vi "Check Protection.vi"(8 "error in (no error)":errorcluster, 10 "String in":string, 11 "LRC - HRZ Series in":refnum<class "LRC - HRZ Series.lvclass">) -> (0 "error out":errorcluster, 1 "Protection Error":errorcluster, 2 "String out":string, 3 "LRC - HRZ Series out":refnum<class "LRC - HRZ Series.lvclass">)   [LabVIEW 2020, in "Protections.lvlib" / "LRC - HRZ Series.lvclass"]
uses:
  LRC - HRZ Series.lvclass
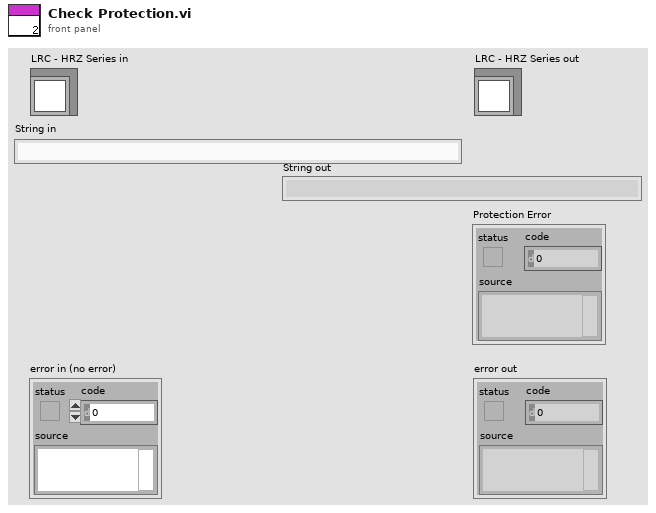
[diagram p1: front panel]
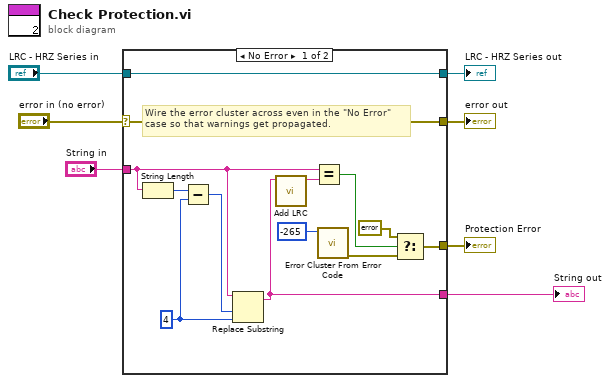
[diagram p0: block diagram]
diagram:
  n1 = case shown="No Error" "error in (no error)" {
    selector: "error in (no error)" -> [w19 w23]
    tunnel: [w19 w23] -> w6
    tunnel: [w20 w22] -> w4
    tunnel: "LRC - HRZ Series in" -> [w20 w22]
    tunnel: "String in" -> [w14 w21]
    tunnel: [w9 _] -> w2
    tunnel: [w8 w21] -> w1
    frame No Error {
      w16 = 4
      # "Wire the error cluster across even in the \"No Error\"\ncase so that warnings get propagated."
      n2 = String Length(string=w14) -> (length=w18:i32)
      n3 = Subtract(x=w18, y=w16) -> (x-y=w17:i32)
      n4 = Replace Substring(2:w16, 3:w17, 5:w14) -> (1:w8:string)  [unwired: 1 in, 1 out]
      n5 = call "Add LRC.vi"("String in"=w8) -> ("String"=w15:string)  [unwired: 9 in, 1 out]
      n6 = Equal?(x=w14, y=w15) -> (x = y?=w10:bool)
      n7 = call <vilib>:"Error Cluster From Error Code.vi"("error code (0)"=-265) -> ("error out"=w13:errorcluster)  [unwired: 8 in]
      n8 = Select(t=errorcluster {"status"=FALSE, "code"=0, "source"=""} ("error in (no error)"), s=w10, f=w13) -> (s? t:f=w9:errorcluster)
    }
    frame Error {
    }
  }
  "error out" <- w6
  "LRC - HRZ Series out" <- w4
  "Protection Error" <- w2
  "String out" <- w1
